vi "macro_SwerveDriveOdomUpdate4.vi"   [LabVIEW 2019, in "Trajectory_Library.lvlib"]
uses:
  Trajectory_Library.lvlib
types:
  T1 = typedef "Trajectory_Library.lvlib/ROTATION2D.ctl" = cluster{"VALUE":dbl, "COS":dbl, "SIN":dbl}
  T2 = typedef "Trajectory_Library.lvlib/SWERVE_DRIVE_MODULE_POSITION.ctl" = cluster{"Distance":dbl, "Angle":T1, "P":bool}
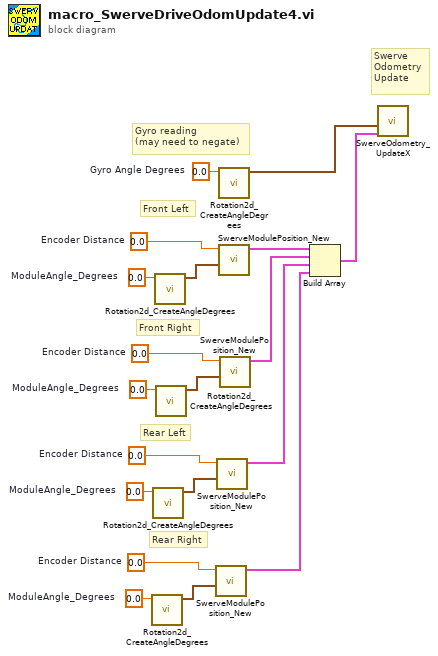
[diagram p0: block diagram]
diagram:
  w6 = 0.0  # ModuleAngle_Degrees
  w8 = 0.0  # Encoder Distance
  w9 = 0.0  # ModuleAngle_Degrees
  w11 = 0.0  # Encoder Distance
  w12 = 0.0  # ModuleAngle_Degrees
  w14 = 0.0  # Encoder Distance
  w16 = 0.0  # Gyro Angle Degrees
  w17 = 0.0  # ModuleAngle_Degrees
  w19 = 0.0  # Encoder Distance
  # "Swerve\nOdometry\nUpdate"
  # "Rear Right"
  # "Rear Left"
  # "Front Right"
  # "Front Left"
  # "Gyro reading\n(may need to negate)"
  n1 = call "Rotation2d_CreateAngleDegrees.vi"("Angle_Degrees"=w6) -> ("ROTATION"=w7:T1)  [unwired: 10 in]
  n2 = call "Rotation2d_CreateAngleDegrees.vi"("Angle_Degrees"=w9) -> ("ROTATION"=w10:T1)  [unwired: 10 in]
  n3 = call "Rotation2d_CreateAngleDegrees.vi"("Angle_Degrees"=w17) -> ("ROTATION"=w18:T1)  [unwired: 10 in]
  n4 = call "Rotation2d_CreateAngleDegrees.vi"("Angle_Degrees"=w12) -> ("ROTATION"=w13:T1)  [unwired: 10 in]
  n5 = call "SwerveModulePosition_New.vi"("ROTATION"=w7, "Distance"=w8) -> ("SWERVE_DRIVE_MODULE_POSITION"=w3:T2)  [unwired: 9 in]
  n6 = call "SwerveModulePosition_New.vi"("ROTATION"=w10, "Distance"=w11) -> ("SWERVE_DRIVE_MODULE_POSITION"=w4:T2)  [unwired: 9 in]
  n7 = call "Rotation2d_CreateAngleDegrees.vi"("Angle_Degrees"=w16) -> ("ROTATION"=w2:T1)  [unwired: 10 in]
  n8 = call "SwerveModulePosition_New.vi"("ROTATION"=w18, "Distance"=w19) -> ("SWERVE_DRIVE_MODULE_POSITION"=w15:T2)  [unwired: 9 in]
  n9 = call "SwerveModulePosition_New.vi"("ROTATION"=w13, "Distance"=w14) -> ("SWERVE_DRIVE_MODULE_POSITION"=w5:T2)  [unwired: 9 in]
  n10 = Build Array(w15, w5, w4, w3) -> (w1:T2[])
  n11 = call "SwerveOdometry_UpdateX.vi"("module Positions"=w1, "gyroAngle"=w2) -> ()  [unwired: 7 in, 3 out]
